vi "Initialize Alarm Time Array.vi"(10 "Alarms Time Array in":T1(array[cluster]), 11 "data":waveform(dbl)[](array[waveform])) -> (3 "Alarms Time Array out":T1(array[cluster]))   [LabVIEW 2018, in "DAQ.lvlib"]
uses:
  DAQ.lvlib
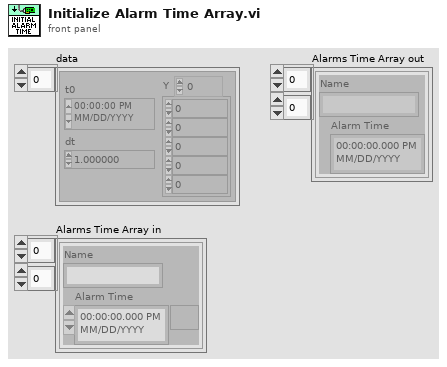
[diagram p1: front panel]
types:
  T1 = cluster{"Name":string, "Alarm Time":timestamp}[][]
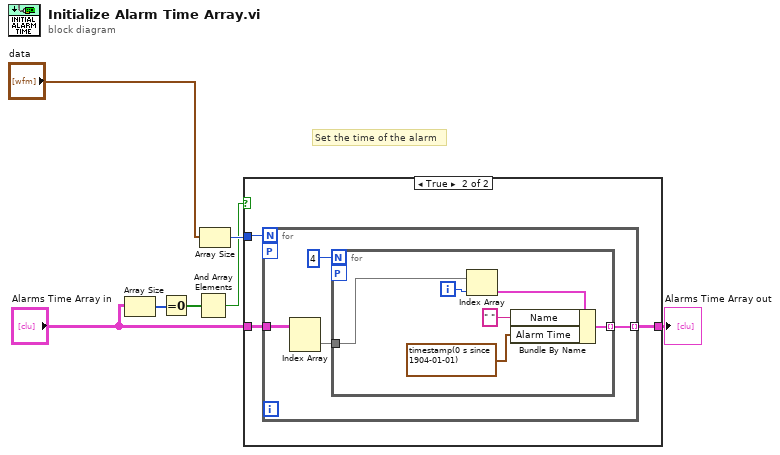
[diagram p0: block diagram]
diagram:
  # "Set the time of the alarm"
  n1 = Array Size(array="Alarms Time Array in") -> (size(s)=w2:i32[])
  n2 = Equal To 0?(x=w2) -> (x = 0?=w3:bool[])
  n3 = And Array Elements(Boolean array=w3) -> (logical AND=w4:bool)
  n4 = Array Size(array="data") -> (size(s)=w5:i32)
  n5 = case shown="True" w4 {
    tunnel: w5 -> [_ w9]
    tunnel: "Alarms Time Array in" -> [w8 w11]
    tunnel: [w8 w10] -> w7
    frame False {
    }
    frame True {
      n6 = for {
        N: w9 -> [_]
        tunnel: w11 -> [w15]
        tunnel: [w13] -> w10 mode=indexing
        workers-P: _ -> [_]
        n7 = Index Array(array=w15) -> (element=w14:cluster{"Name":string, "Alarm Time":timestamp}[])  [unwired: 2 in]
        n8 = for {
          N: 4 -> [_]
          tunnel: [w19] -> w13 mode=indexing
          tunnel: w14 -> [w18]
          workers-P: _ -> [_]
          i -> [w17]
          n9 = Index Array(array=w18, index=w17) -> (element=w16:cluster{"Name":string, "Alarm Time":timestamp})
          n10 = Bundle By Name(cluster=w16, "Name"=" ", "Alarm Time"=timestamp(0 s since 1904-01-01)) -> (w19:cluster{"Name":string, "Alarm Time":timestamp})
        }
      }
    }
  }
  "Alarms Time Array out" <- w7
